vi "Fetch Multi Eval Meas ES Flatness Subcarrier Index Results.vi"(8 "error in (no error)":errorcluster, 10 "Instance (1)":T2=1, 11 "VISA resource name":refnum<visa-resource-name>) -> (0 "error out":errorcluster, 1 "ES Flatness Subcarrier Index Results":T1 {"Out Of Tolerance" format="%^.3e"}, 2 "Reliability":i32, 3 "VISA resource name out":refnum<visa-resource-name>)   [LabVIEW 2020, in "Rohde&Schwarz CMXP NR FR2 Measurement.lvlib"]
doc: "Returns subcarrier indices of the multi eval measurement ES Flatness results.\n\nAttribute:\nRSCMXPNRFR2M_ATTR_FETCH_MULTI_EVAL_MEASUREMENT_ESF_SCINDEX_RESULTS\n\nRemote-control command:\nFETCh:NRMMw:MEAS<i>:MEValuation:ESFLatness:CURRent:SCINdex?"
uses:
  <instrlib>/Rohde&Schwarz CMXP NR FR2 Measurement/Rohde&Schwarz CMXP NR FR2 Measurement.lvlib
  <instrlib>/Rohde&Schwarz CMXP NR FR2 Measurement/Private/_Instance.ctl
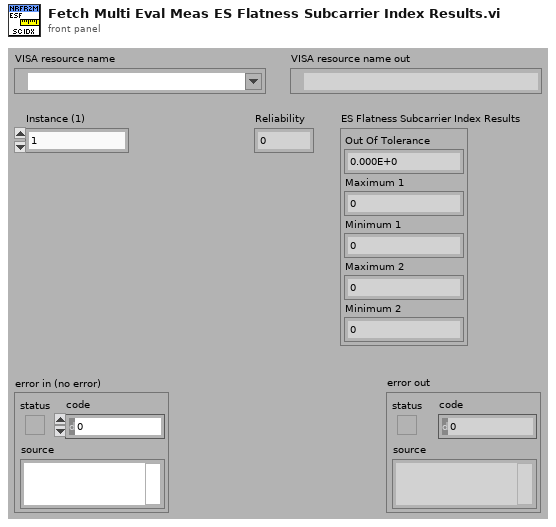
[diagram p1: front panel]
types:
  T1 = cluster{"Out Of Tolerance":dbl, "Maximum 1":i32, "Minimum 1":i32, "Maximum 2":i32, "Minimum 2":i32}
  T2 = typedef "Rohde&Schwarz CMXP NR FR2 Measurement.lvlib/_Instance.ctl" = i32
  T3 = cluster{"Out Of Tolerance":dbl, "Val 1":i32, "Val 2":i32, "Val 3":i32, "Val 4":i32}
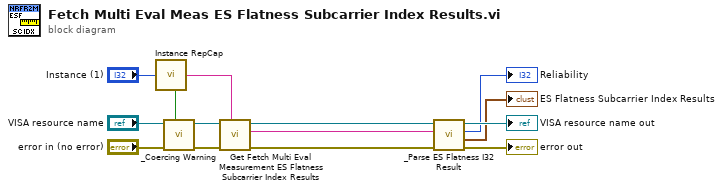
[diagram p0: block diagram]
diagram:
  n1 = call <instrlib>:"Instance RepCap.vi"("Instance In"="Instance (1)") -> ("In Range?"=w3:bool, "RepCap Identifier Out"=w14:string)  [unwired: 1 in]
  n2 = call <instrlib>:"_Coercing Warning.vi"("In Range?"=w3, "error in (no error)"="error in (no error)", "VISA resource name"="VISA resource name") -> ("error out"=w4:errorcluster, "VISA resource name out"=w5:refnum<visa-resource-name>)  [unwired: 7 in]
  n3 = call "Get Fetch Multi Eval Measurement ES Flatness Subcarrier Index Results"("Repeated Capabilities"=w14, "error in (no error)"=w4, "instrument handle"=w5) -> ("error out"=w13:errorcluster, "Fetch Multi Eval Measurement ES Flatness Subcarrier Index Results"=w8:string, "instrument handle out"=w12:refnum<visa-resource-name>)  [unwired: 6 in]
  n4 = call <instrlib>:"_Parse ES Flatness I32 Result.vi"("error in (no error)"=w13, "Input String"=w8, "VISA resource name"=w12) -> ("error out"=→"error out":errorcluster, "Result"=→"ES Flatness Subcarrier Index Results":T3, "Reliability"=→"Reliability":i32, "VISA resource name out"=→"VISA resource name out":refnum<visa-resource-name>)  [unwired: 5 in]
